vi "Ej 8 String_Concatenado.vi"() -> ()   [LabVIEW 2021]
panel:
  out "OUTPUT":dbl
  out "before substring":string
  out "after substring":string
  out "match substring":string
  out "offset past match":i32
  in  "INPUT":dbl
  out "Longitud":i32
  in  "Unidades":string
  in  "Encabezado":string="El valor del voltaje es:"
  out "Concatenacion":string
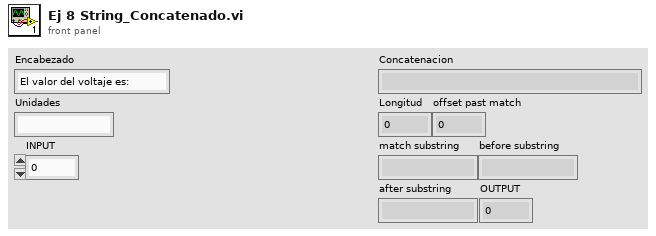
[diagram p1: front panel]
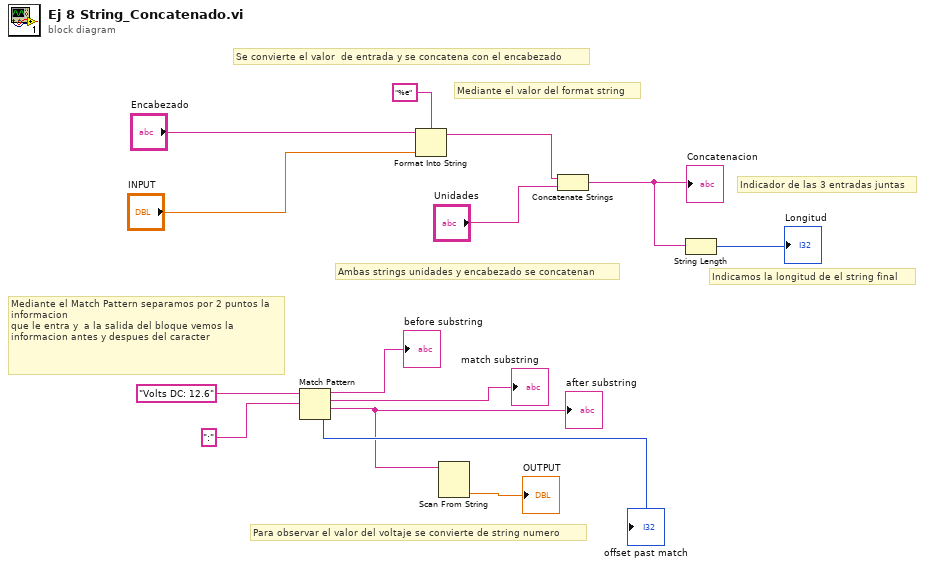
[diagram p0: block diagram]
diagram:
  # "Mediante el Match Pattern separamos por 2 puntos la informacion\nque le entra y  a la salida del bloque vemos la informacion antes y despues del caracter"
  # "Mediante el valor del format string"
  # "Indicamos la longitud de el string final"
  # "Indicador de las 3 entradas juntas"
  # "Ambas strings unidades y encabezado se concatenan"
  # "Se convierte el valor  de entrada y se concatena con el encabezado"
  # "Para observar el valor del voltaje se convierte de string numero"
  n1 = Match Pattern(string="Volts DC: 12.6", regular expression=":") -> (before substring=→"before substring":string, match substring=→"match substring":string, after substring=w1:string, offset past match=→"offset past match":i32)  [unwired: 1 in]
  "after substring" <- w1
  n2 = Format Into String "Format Into String"(format string="%e", initial string="Encabezado", "INPUT") -> (resulting string=w13:string)  [unwired: 1 in, 1 out]
  n3 = Scan From String "Scan From String"(input string=w1) -> (output 1=→"OUTPUT":dbl)  [unwired: 4 in, 3 out]
  n4 = Concatenate Strings "Concatenate Strings"(w13, "Unidades") -> (w12:string)
  "Concatenacion" <- w12
  n5 = String Length(string=w12) -> (length=→"Longitud":i32)
